vi "Get Interface.vi"(11 "Plugin in":refnum<class "Dispatcher Thread.lvclass">) -> (2 "Interface":refnum<class "Dispatcher Interface.lvclass">, 3 "Plugin out":refnum<class "Dispatcher Thread.lvclass">)   [LabVIEW 2017, in "DSF Core.lvlib" / "Dispatcher Thread.lvclass"]
uses:
  Dispatcher Thread.lvclass
  Interface/Dispatcher/Dispatcher Interface.lvclass
  Dispatcher Thread.lvclass/Dispatcher Thread.ctl
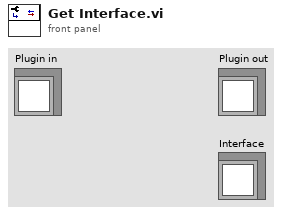
[diagram p1: front panel]
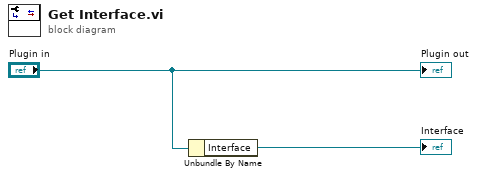
[diagram p0: block diagram]
diagram:
  n1 = Unbundle By Name("Plugin in") -> ("Interface"=→"Interface":refnum<class "Dispatcher Interface.lvclass">)
  "Plugin out" <- "Plugin in"
